vi "CSM User Interface(UI) Module Template.vi"(7 "Name (\"\" to Use UUID)":string="Event CSM") -> ()   [LabVIEW 2017]
doc: "A template for creating a CSM module with a user interface. This template includes a user Event Structure for responding to user actions.\n\n\n> [!NOTE] <b>CSM Naming Rules</b>\n>\n> - CSM module name must be unique. Otherwise, CSM enters a `Critical Error` state.\n> - If the input module name is an empty string (\"\"), the system uses a UUID as the module name. Such a module is marked as standalone mode and does not appear in the module list.\n> - Worker Mode Rule: If the input module name ends with `#`, a worker mode node will be instantiated. Multiple worker mode nodes can form a worker mode module.\n> - Chain of Responsibility Mode Rule: If the input module name ends with `$` followed by a number, a chain of responsibility mode node will be instantiated. Multiple chain of responsibility mode nodes can form a chain of responsibility mode module. Smaller numbers mean higher priority, and messages are routed directly to the highest-priority node that can handle them.\n> - System-Level Module Rule: If the input module name starts with `.`, the module is a system-level module. Under default settings, such modules are not listed by the CSM - List Modules VI and are suitable for instantiating modules that run in the background.\n> - Submodule Rule: `.` is also allowed in a module name to separate the module name into multiple parts. CSM does not have strict rules for submodules. The `.` in the module name only marks the logical relationship between different modules. From an execution perspective, they are considered independent modules. The only difference is that you can obtain a list of logical submodules via the CSM - List Submodules VI.\n\n\n> [!NOTE] <b>CSM Initialize State (\"Macro: Initialize\")</b>\n>\n> - The default value is `Macro: Initialize`, which is consistent with the JKISM state machine.\n> - This state is used to initialize the state machine of a CSM module. A CSM module will process externally sent messages only after completing this macro state.\n\n\n> [!NOTE] <b>CSM Exit State (\"Macro: Exit\")</b>\n>\n> - The default value is \"Macro: Exit\", which is consistent with the JKISM state machine.\n> - This state is used to exit the state machine of a CSM module. After entering this state, a CSM module no longer processes externally sent messages.\n\n\n> [!WARNING] <b>Multiple CSMs in a Single VI</b>\n>\n> - It is not recommended to place multiple (>=2) CSMs in a flat layout within a single VI. While this will not cause logical issues in the program, it will prevent the CSM Debug Console from loading all the inner and outer interfaces of the flat CSMs in that VI - only one will be loaded.\n\n\n-- <b>Controls</b> --\n- <b>Name (\"\" to use UUID)</b>: CSM module name. Refer to <b>CSM Naming Rules</b> for module naming rules."
uses:
  AdvanceAPI/CSM - Revert Arguments-Safe String.vi
  _Shared/Trim Single-line Text.vi
  AdvanceAPI/CSM - Break Down Multiple States String.vi
  AdvanceAPI/CSM - Compact Multiple States.vi
  AdvanceAPI/CSM - Make String Arguments Safe.vi
  AdvanceAPI/CSM - Keywords.vi
  Communicable State Machine.lvlib
panel:
  out "State History":string
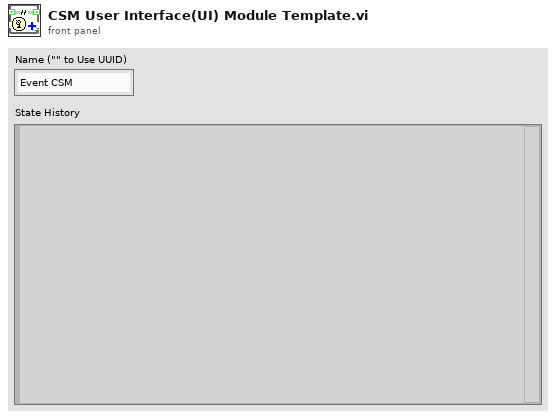
[diagram p1: front panel]
types:
  T1 = enum32{"Invalid", "Standard", "Closed", "Hidden", "Minimized", "Maximized"}
  T2 = enum32{"invalid app kind", "Development System", "Run Time System", "Student Edition", "Embedded LabVIEW", "Evaluation", "Custom"}
  T3 = typedef "Communicable State Machine.lvlib/_CSM_Response Source Message.ctl" = cluster{"‘State":string, "’Arguments":string, "’Error":errorcluster}
  T4 = cluster{"Current VI Reference":refnum<vi>, "Close Panel on Exit?":bool}
  T5 = cluster{"Core":cluster{"Current VI Reference":refnum<vi>, "Close Panel on Exit?":bool}, "Your Boolean data":bool, "Your string data":string}
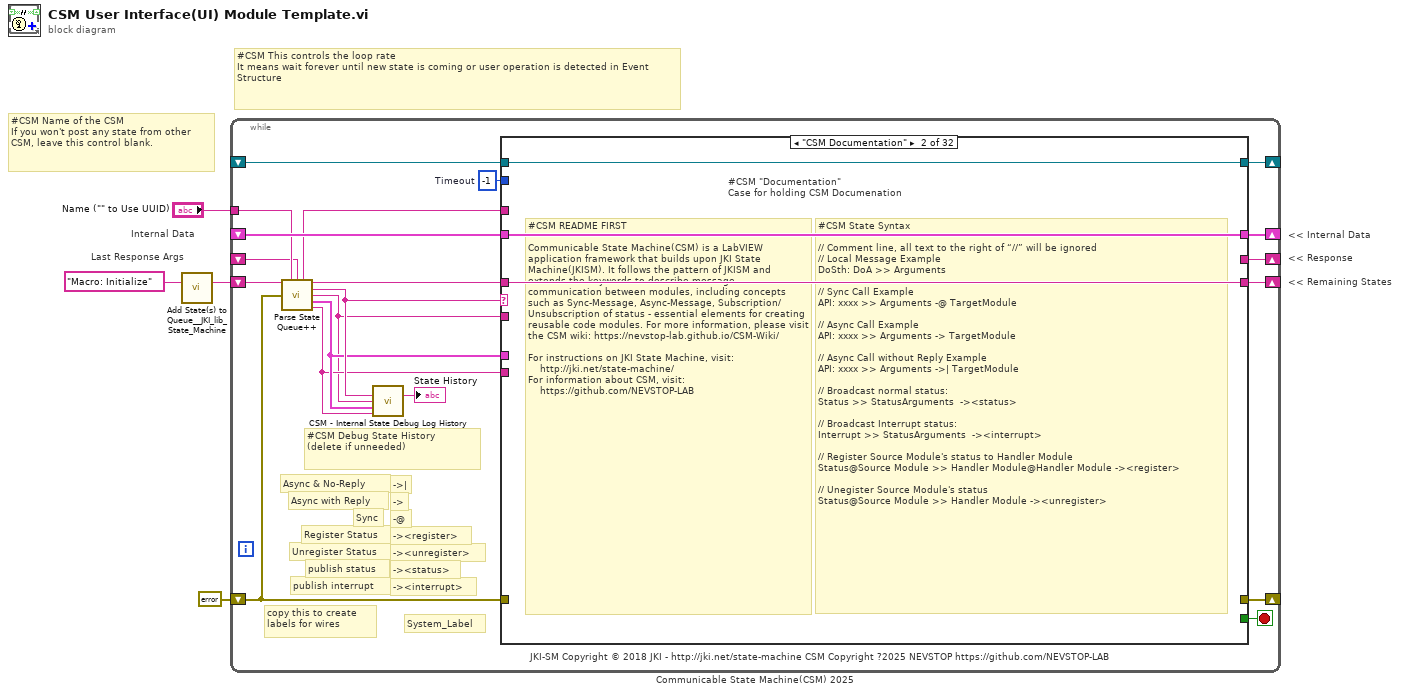
[diagram p0: block diagram]
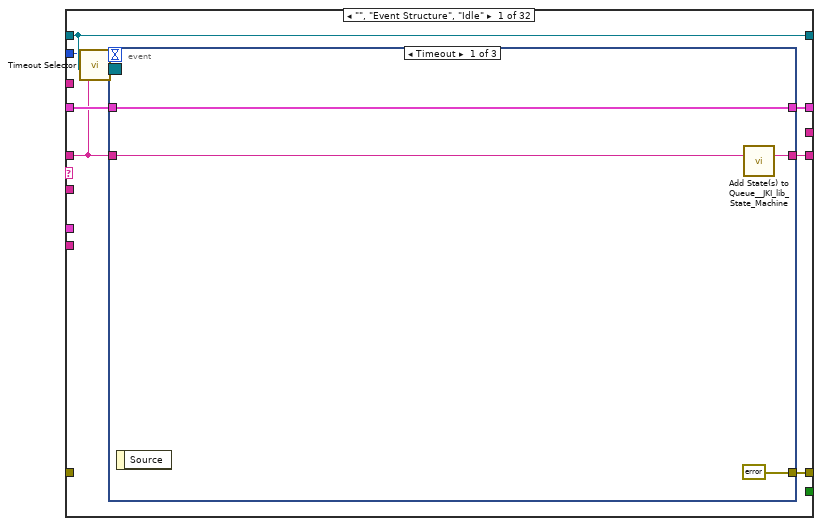
[diagram p2: hidden frame]
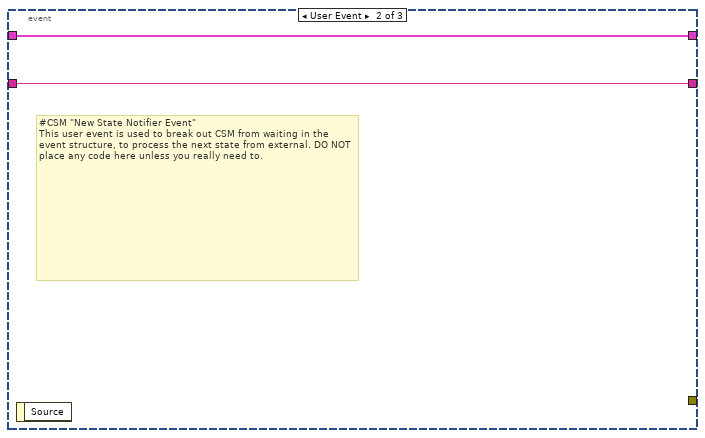
[diagram p3: hidden frame]
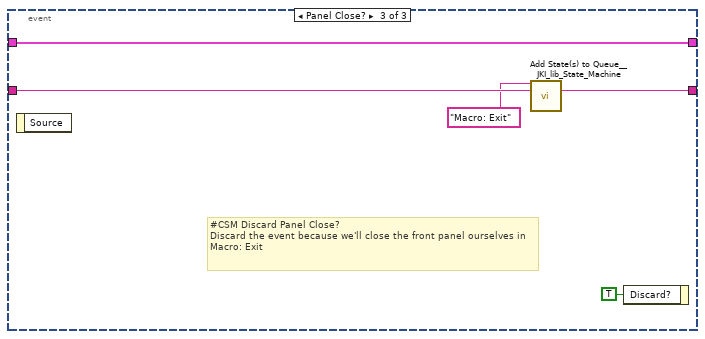
[diagram p4: hidden frame]
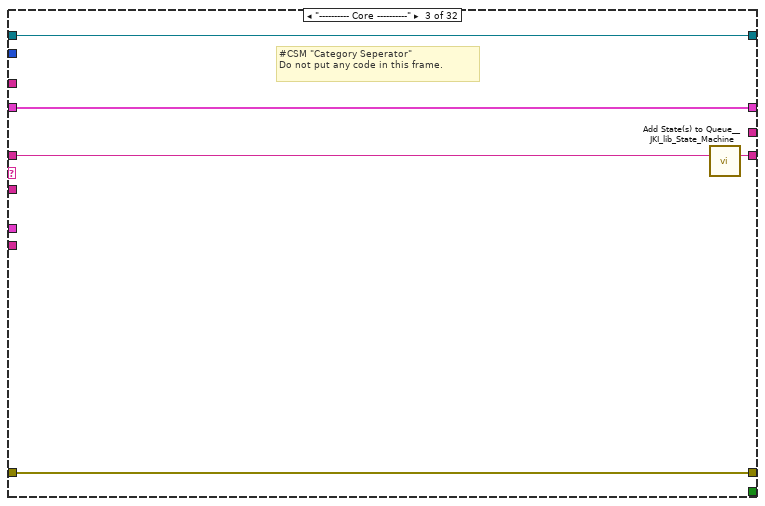
[diagram p5: hidden frame]
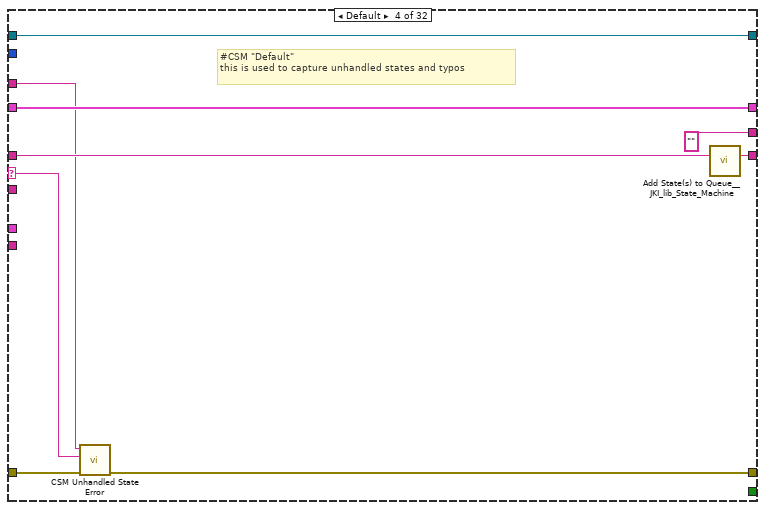
[diagram p6: hidden frame]
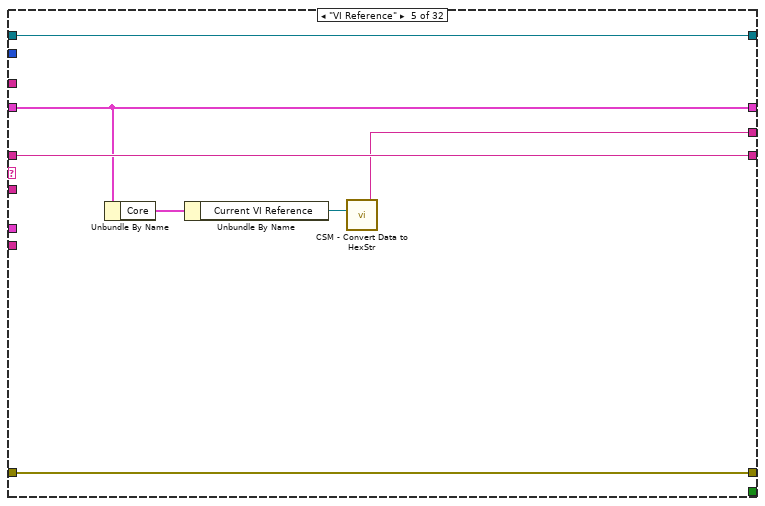
[diagram p7: hidden frame]
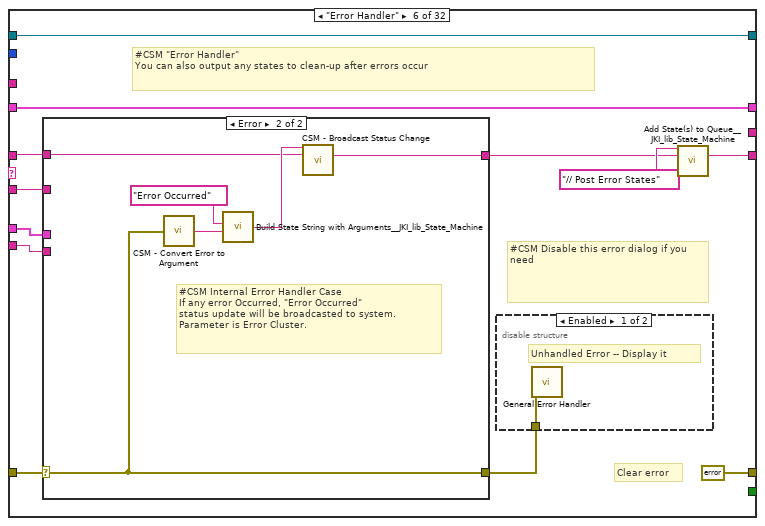
[diagram p8: hidden frame]
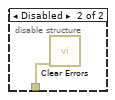
[diagram p9: hidden frame]
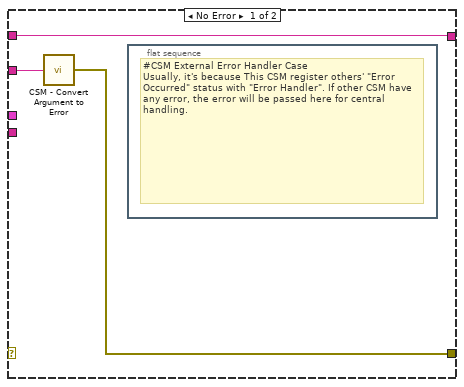
[diagram p10: hidden frame]
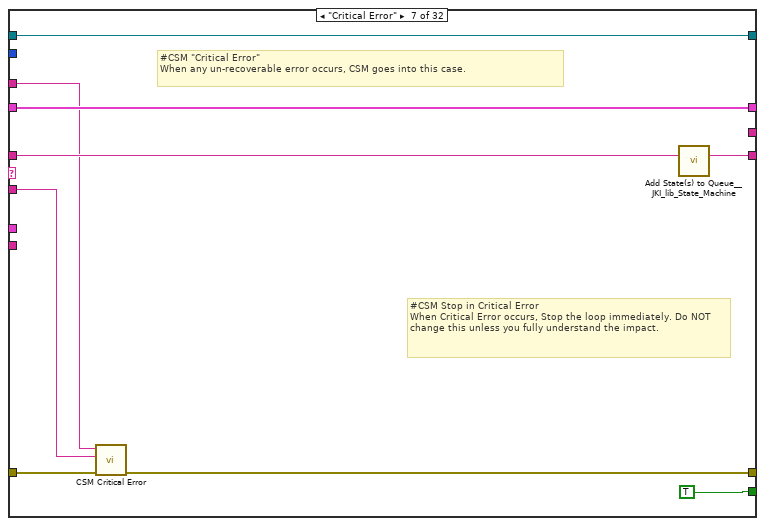
[diagram p11: hidden frame]
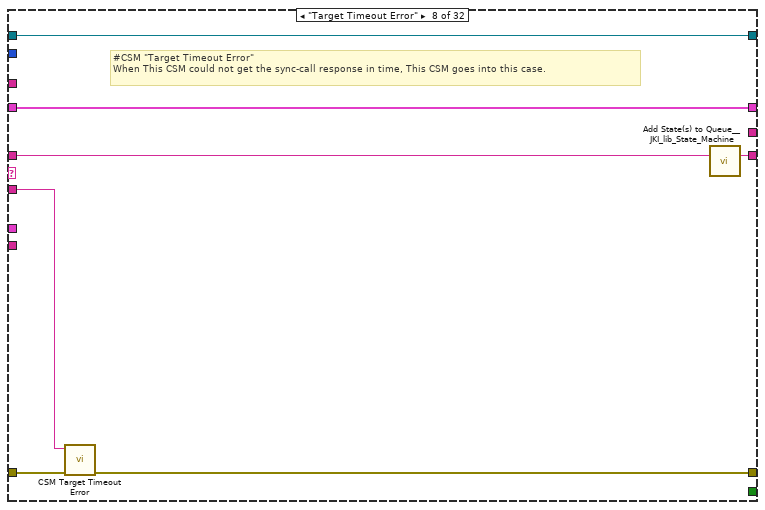
[diagram p12: hidden frame]
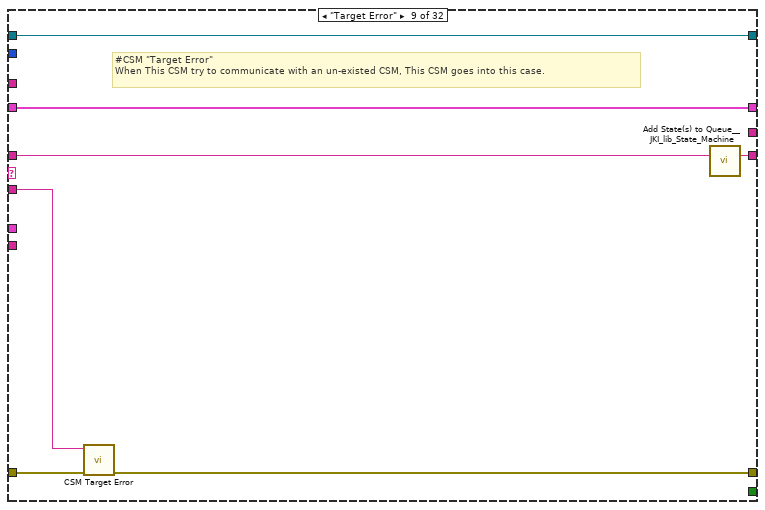
[diagram p13: hidden frame]
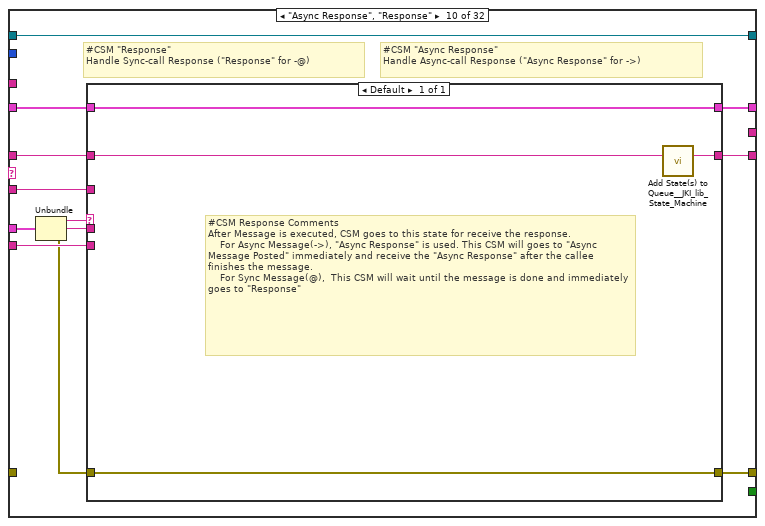
[diagram p14: hidden frame]
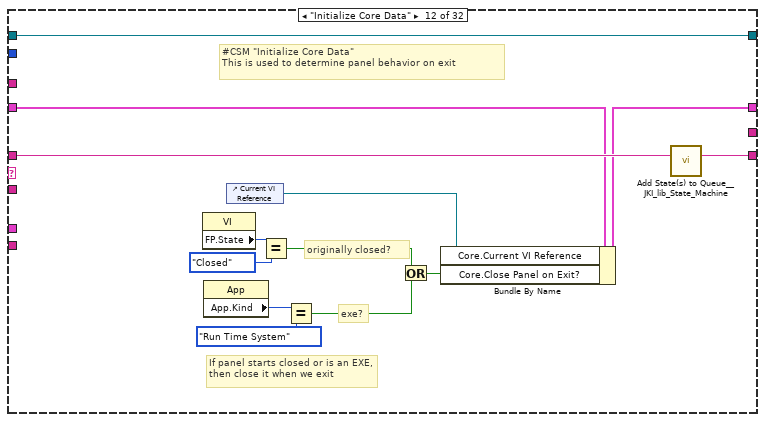
[diagram p16: hidden frame]
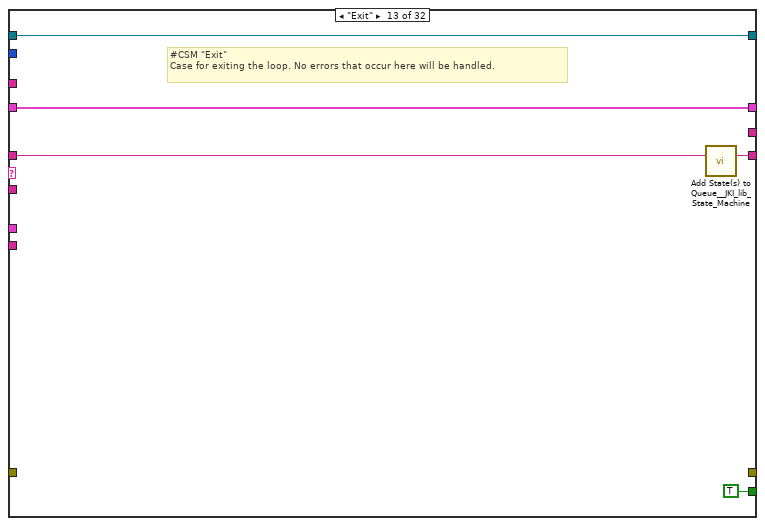
[diagram p17: hidden frame]
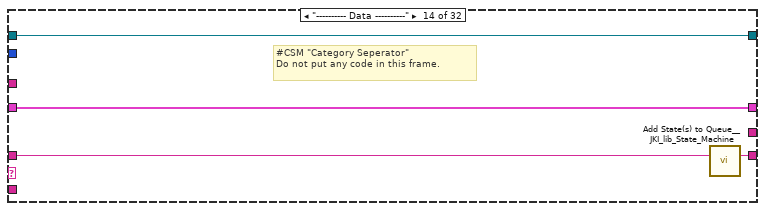
[diagram p18: hidden frame]
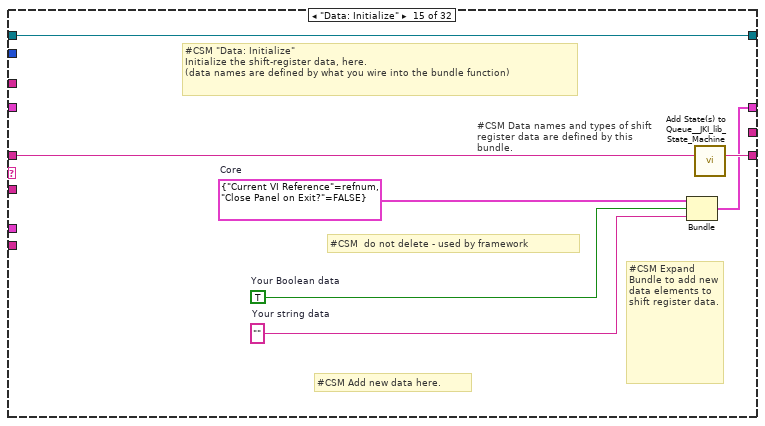
[diagram p19: hidden frame]
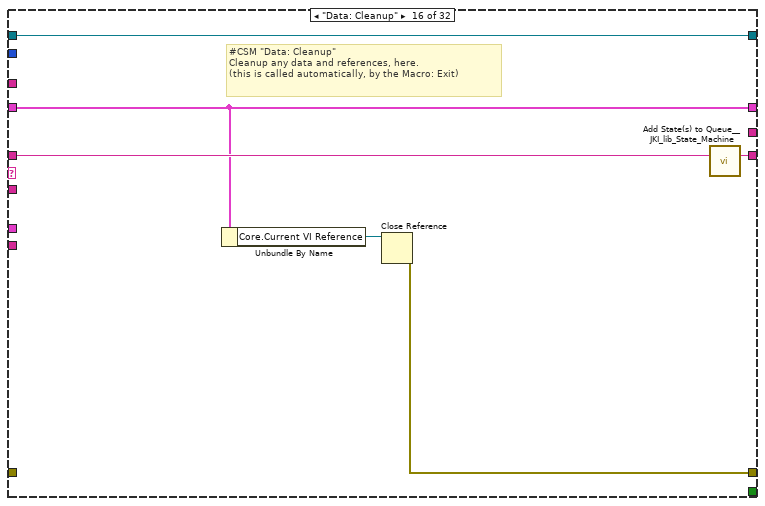
[diagram p20: hidden frame]
diagram:
  # "Last Response Args"
  # "Internal Data"
  # "<< Internal Data"
  # "<< Response"
  # "<< Remaining States"
  # "#CSM Name of the CSM\nIf you won't post any state from other CSM, leave this control blank."
  # "#CSM This controls the loop rate\nIt means wait forever until new state is coming or user operation is detected in Event Structure"
  n1 = call <vilib>:"Add State(s) to Queue__JKI_lib_State_Machine.vi"("State(s) in (\"\")"="Macro: Initialize" ("Init State(\"Macro: Initialize\")")) -> ("States Out"=w4:string)  [unwired: 14 in]
  n2 = while "Communicable State Machine(CSM) 2025" {
    shift-right: [w19] -> _
    shift-left: _ -> [w18]
    shift-right: [w22] -> _
    shift-left: errorcluster {"status"=FALSE, "code"=0, "source"=""} ("error out") -> [w16]
    shift-right: [w21] -> _
    shift-left: w4 -> [w23]
    tunnel: "Name (\"\" to Use UUID)" -> [w12]
    shift-right: [w15] -> _
    shift-left: _ -> [w7]
    shift-right: [w14] -> _
    shift-left: _ -> [w13]
    stop <- w20 stop-if-true
    w17 = -1  # Timeout
    # "#CSM Debug State History\n(delete if unneeded)"
    # "-><interrupt>"
    # "-><status>"
    # "-><unregister>"
    # "-><register>"
    # "-@"
    # "->"
    # "->|"
    # "publish interrupt"
    # "publish status"
    # "Unregister Status"
    # "Register Status"
    # "Sync"
    # "Async with Reply"
    # "Async & No-Reply"
    # "copy this to create labels for wires"
    # "System_Label"
    # "JKI-SM Copyright © 2018 JKI - http://jki.net/state-machine CSM Copyright ?2025 NEVSTOP https://github.com/NEVSTOP-LAB"
    n3 = call "Parse State Queue++.vi"("State Queue"=w23, "Name (\"\" to Use UUID)"=w12, "Response Arguments"=w7, "Previous Error"=w16) -> ("Name Used"=w8:string, "Remaining States"=w24:string, "Current State"=w11:string, "Arguments"=w6:string, "Additional Information"=w10:T3, "Source CSM"=w9:string)  [unwired: 6 in]
    n4 = call "CSM - Internal State Debug Log History.vi"("State"=w11, "Arguments (\"\")"=w6, ">> Response Source Message >>"=w10, "Source (\"\")"=w9) -> ("Debug Log"=→"State History":string)  [unwired: 11 in]
    n5 = case shown="\"CSM Documentation\"" w11 {
      selector: w11 -> [_ _ _ w54 _ _ _ _ _ _ _ _ _ _ _ _ _ _ _ _ _ _ _ _ _ _ _ _ _ _ _ _]
      tunnel: w24 -> [w25 w46 w51 w60 w66 w72 w98 w106 w113 w123 w132 w145 w150 w154 w161 w167 w171 w178 w182 w186 w190 w196 w207 w271 w276 w287 w290 w294 w297 w301 w305 w309]
      tunnel: w6 -> [_ _ _ _ _ w70 w94 w101 w109 w117 _ _ _ _ _ _ _ _ _ _ _ w192 w202 _ _ _ _ _ _ _ _ _]
      tunnel: w18 -> [w31 w45 w48 w58 w65 w78 w99 w104 w111 w121 w131 w139 w148 w152 _ w163 w169 w177 w181 w184 w188 w194 w204 w269 w274 w285 w289 w293 w296 w299 w303 w307]
      tunnel: [w30 _ w49 w52 w67 errorcluster {"status"=FALSE, "code"=0, "source"=""} ("error out") w91 w100 w107 w120 _ _ _ _ _ w164 _ w172 w180 _ _ w193 w205 _ _ _ _ _ _ _ _ _] -> w22
      tunnel: w16 -> [_ _ w49 w53 w67 w76 w92 w102 w108 _ _ _ _ _ _ _ _ _ _ _ _ _ _ _ _ _ _ _ _ _ _ _]
      tunnel: [w32 w46 w50 w59 w66 w74 w97 w105 w112 w124 w132 w144 w149 w153 w160 w166 w170 w178 w182 w185 w189 w195 w206 w270 w275 w286 w290 w294 w297 w300 w304 w308] -> w21
      tunnel: [_ _ _ _ _ _ TRUE _ _ _ _ _ TRUE _ _ _ _ _ _ _ _ _ _ _ _ _ _ _ _ _ _ _] -> w20
      tunnel: [w29 w45 w48 w58 w65 w78 w99 w104 w111 w122 w131 w143 w148 w152 w159 w163 w169 w177 w181 w184 w188 w194 w204 w269 w274 w285 w289 w293 w296 w299 w303 w307] -> w19
      tunnel: w17 -> [w27 _ _ _ _ _ _ _ _ _ _ _ _ _ _ _ _ _ _ _ _ _ _ _ _ _ _ _ _ _ _ _]
      tunnel: w9 -> [_ _ _ _ _ w69 _ _ _ w118 _ _ _ _ _ _ _ _ _ _ _ _ _ _ _ _ _ _ _ _ _ _]
      tunnel: w10 -> [_ _ _ _ _ w68 _ _ _ w119 _ _ _ _ _ _ _ _ _ _ _ _ _ _ _ _ _ _ _ _ _ _]
      tunnel: [_ _ _ "" w61 _ _ _ _ _ _ _ _ _ _ _ _ _ _ _ _ _ _ _ _ _ _ "API1 Response" _ _ _ _] -> w15
      tunnel: [w28 w44 w47 w56 w64 w77 w95 w103 w110 w125 w130 w133 w146 w151 w155 w162 w168 w176 w179 w183 w187 w191 w201 w268 w272 w278 w288 w292 w295 w298 w302 w306] -> w14
      tunnel: w13 -> [w28 w44 w47 w56 w64 w77 w95 w103 w110 w125 w130 w133 w146 w151 w155 w162 w168 _ w179 w183 w187 w191 w201 w268 w272 w278 w288 w292 w295 w298 w302 w306]
      tunnel: w8 -> [_ _ _ w55 _ _ w93 _ _ _ _ _ _ _ _ _ _ w175 _ _ _ _ _ _ _ _ _ _ _ _ _ _]
      frame "", "Event Structure", "Idle" {
        n6 = call "Timeout Selector.vi"("Remaining States"=w25, "Timeout Expected"=w27) -> ("Timeout"=w26:i32)  [unwired: 5 in]
        n7 = event shown="[0] Timeout" {
          selector: w28 -> [_ _ _]
          dyn-events: _ -> [_ _ _]
          timeout: w26 -> [_ _ _]
          tunnel: w25 -> [w36 w37 w43]
          tunnel: [w35 w37 w42] -> w32
          tunnel: w31 -> [w34 w38 w41]
          tunnel: [errorcluster {"status"=FALSE, "code"=0, "source"=""} ("error out") _ _] -> w30
          tunnel: [w34 w38 w41] -> w29
          event Timeout {
            n8 = event-data() -> ()  [unwired: 1 in, 1 out]
            n9 = call <vilib>:"Add State(s) to Queue__JKI_lib_State_Machine.vi"("State(s) in (\"\")"=w36) -> ("States Out"=w35:string)  [unwired: 14 in]
          }
          event User Event {
            # "#CSM \"New State Notifier Event\"\nThis user event is used to break out CSM from waiting in the event structure, to process the next state from external. DO NOT place any code here unless you really need to."
            n10 = event-data() -> ()  [unwired: 1 in, 1 out]
          }
          event Panel Close? {
            # "#CSM Discard Panel Close?\nDiscard the event because we'll close the front panel ourselves in Macro: Exit"
            n11 = event-data() -> ()  [unwired: 1 in, 1 out]
            n12 = call <vilib>:"Add State(s) to Queue__JKI_lib_State_Machine.vi"("State(s) in Front (\"\")"="Macro: Exit", "State(s) in (\"\")"=w43) -> ("States Out"=w42:string)  [unwired: 13 in]
            n13 = event-data("Discard?"=TRUE) -> ()  [unwired: 1 in, 1 out]
          }
        }
      }
      frame "CSM Documentation" {
        # "#CSM State Syntax\n\n// Comment line, all text to the right of “//” will be ignored\n// Local Message Example\nDoSth: DoA >> Arguments\n\n// Sync Call Example\nAPI: xxxx >> Arguments -@ TargetModule\n\n// Async Call Example\nAPI: xxxx >> Arguments -> TargetModule\n\n// Async Call without Reply Example\nAPI: xxxx >> Arguments ->| TargetModule\n\n// Broadcast normal status:\nStatus >> StatusArguments  -><status>\n\n// Broadcast Interrupt status:\nInterrupt >> StatusArguments  -><interrupt>\n\n// Register Source Module's status to Handler Module\nStatus@Source Module >> Handler Module@Handler Module -><register>\n\n// Unegister Source Module's status\nStatus@Source Module >> Handler Module -><unregister>"
        # "#CSM README FIRST\n\nCommunicable State Machine(CSM) is a LabVIEW application framework that builds upon JKI State Machine(JKISM). It follows the pattern of JKISM and extends the keywords to describe message communication between modules, including concepts such as Sync-Message, Async-Message, Subscription/Unsubscription of status - essential elements for creating reusable code modules. For more information, please visit the CSM wiki: https://nevstop-lab.github.io/CSM-Wiki/\n\nFor instructions on JKI State Machine, visit: \n    http://jki.net/state-machine/\nFor information about CSM, visit: \n    https://github.com/NEVSTOP-LAB"
        # "#CSM \"Documentation\"\nCase for holding CSM Documenation"
      }
      frame "---------- Core ----------" {
        # "#CSM \"Category Seperator\"\nDo not put any code in this frame."
        n14 = call <vilib>:"Add State(s) to Queue__JKI_lib_State_Machine.vi"("State(s) in (\"\")"=w51) -> ("States Out"=w50:string)  [unwired: 14 in]
      }
      frame Default {
        # "#CSM \"Default\"\nthis is used to capture unhandled states and typos"
        n15 = call "CSM Unhandled State Error.vi"("error in (no error)"=w53, "Undefined State"=w54, "CSM Name"=w55) -> ("error out"=w52:errorcluster)  [unwired: 8 in]
        n16 = call <vilib>:"Add State(s) to Queue__JKI_lib_State_Machine.vi"("State(s) in (\"\")"=w60) -> ("States Out"=w59:string)  [unwired: 14 in]
      }
      frame "VI Reference" {
        n17 = Unbundle By Name(w65) -> ("Core"=w63:T4)
        n18 = Unbundle By Name(w63) -> ("Current VI Reference"=w62:refnum<vi>)
        n19 = call "CSM - Convert Data to HexStr.vi"("Variant"=w62) -> ("HEX String (0-9,A-F)"=w61:string)  [unwired: 8 in]
      }
      frame "Error Handler" {
        # "#CSM Disable this error dialog if you need"
        # "#CSM \"Error Handler\"\nYou can also output any states to clean-up after errors occur"
        # "Clear error"
        n20 = case shown="Error" w76 {
          selector: w76 -> [_ w85]
          tunnel: [w83 w87] -> w73
          tunnel: w72 -> [w83 w86]
          tunnel: [w82 w85] -> w71
          tunnel: w70 -> [w84 _]
          tunnel: w69 -> [_ _]
          tunnel: w68 -> [_ _]
          frame No Error {
            n21 = call "CSM - Convert Argument to Error.vi"("Argument"=w84) -> ("Error"=w82:errorcluster)  [unwired: 4 in]
            n22 = flat-sequence {
              frame #0 {
                # "#CSM External Error Handler Case\nUsually, it's because This CSM register others' \"Error Occurred\" status with \"Error Handler\". If other CSM have any error, the error will be passed here for central handling."
              }
            }
          }
          frame Error {
            # "#CSM Internal Error Handler Case \nIf any error Occurred, \"Error Occurred\" \nstatus update will be broadcasted to system.\nParameter is Error Cluster."
            n23 = call "CSM - Convert Error to Argument.vi"("Error"=w85) -> ("Argument"=w89:string)  [unwired: 4 in]
            n24 = call <vilib>:"Build State String with Arguments__JKI_lib_State_Machine.vi"("Arguments (\"\")"=w89, "State"="Error Occurred" ("Status with Arguments")) -> ("State with Arguments"=w88:string)  [unwired: 4 in]
            n25 = call "CSM - Broadcast Status Change.vi"("Status With Arguments"=w88, "State Queue"=w86) -> ("Remaining States"=w87:string)  [unwired: 13 in]
          }
        }
        n26 = disable-structure shown="Enabled" {
          disable-tunnel: w71 -> [w80 w81]
          frame Enabled {
            # "Unhandled Error -- Display it"
            n27 = call <vilib>:"General Error Handler.vi"("error in (no error)"=w80) -> ()  [unwired: 10 in, 5 out]
          }
          frame Disabled {
            n28 = call <vilib>:"Clear Errors.vi"("error in (no error)"=w81) -> ()  [unwired: 5 in, 2 out]
          }
        }
        n29 = call <vilib>:"Add State(s) to Queue__JKI_lib_State_Machine.vi"("State(s) in Front (\"\")"="// Post Error States", "State(s) in (\"\")"=w73) -> ("States Out"=w74:string)  [unwired: 13 in]
      }
      frame "Critical Error" {
        # "#CSM \"Critical Error\"\nWhen any un-recoverable error occurs, CSM goes into this case."
        # "#CSM Stop in Critical Error\nWhen Critical Error occurs, Stop the loop immediately. Do NOT change this unless you fully understand the impact."
        n30 = call "CSM Critical Error.vi"("error in (no error)"=w92, "Arugments (As Reason)"=w94, "CSM Name"=w93) -> ("error out"=w91:errorcluster)  [unwired: 8 in]
        n31 = call <vilib>:"Add State(s) to Queue__JKI_lib_State_Machine.vi"("State(s) in (\"\")"=w98) -> ("States Out"=w97:string)  [unwired: 14 in]
      }
      frame "Target Timeout Error" {
        # "#CSM \"Target Timeout Error\"\nWhen This CSM could not get the sync-call response in time, This CSM goes into this case."
        n32 = call "CSM Target Timeout Error.vi"("error in (no error)"=w102, "Arguments (As CSM Name)"=w101) -> ("error out"=w100:errorcluster)  [unwired: 9 in]
        n33 = call <vilib>:"Add State(s) to Queue__JKI_lib_State_Machine.vi"("State(s) in (\"\")"=w106) -> ("States Out"=w105:string)  [unwired: 14 in]
      }
      frame "Target Error" {
        # "#CSM \"Target Error\"\nWhen This CSM try to communicate with an un-existed CSM, This CSM goes into this case."
        n34 = call "CSM Target Error.vi"("error in (no error)"=w108, "Arguments (As CSM Name)"=w109) -> ("error out"=w107:errorcluster)  [unwired: 9 in]
        n35 = call <vilib>:"Add State(s) to Queue__JKI_lib_State_Machine.vi"("State(s) in (\"\")"=w113) -> ("States Out"=w112:string)  [unwired: 14 in]
      }
      frame "Async Response", "Response" {
        # "#CSM \"Async Response\"\nHandle Async-call Response (\"Async Response\" for ->)"
        # "#CSM \"Response\"\nHandle Sync-call Response (\"Response\" for -@)"
        n36 = Unbundle(w119) -> ("‘State"=w116:string, "’Arguments"=w115:string, "’Error"=w114:errorcluster)
        n37 = case shown="Default" w116 {
          tunnel: [w126] -> w124
          tunnel: w123 -> [w127]
          tunnel: [w129] -> w122
          tunnel: w121 -> [w129]
          tunnel: [w128] -> w120
          tunnel: w114 -> [w128]
          tunnel: w118 -> [_]
          tunnel: w117 -> [_]
          tunnel: w115 -> [_]
          frame Default {
            # "#CSM Response Comments\nAfter Message is executed, CSM goes to this state for receive the response.\n    For Async Message(->), \"Async Response\" is used. This CSM will goes to \"Async Message Posted\" immediately and receive the \"Async Response\" after the callee finishes the message.\n    For Sync Message(@),  This CSM will wait until the message is done and immediately goes to \"Response\""
            n38 = call <vilib>:"Add State(s) to Queue__JKI_lib_State_Machine.vi"("State(s) in (\"\")"=w127) -> ("States Out"=w126:string)  [unwired: 14 in]
          }
        }
      }
      frame "Async Message Posted" {
        # "#CSM \"Async Message Posted\"\nAfter Async Message is posted (-> or ->| ), CSM goes to this state for post-action.\nYou can use Argument - State to tell which Async Message is called."
      }
      frame "Initialize Core Data" {
        # "#CSM \"Initialize Core Data\"\nThis is used to determine panel behavior on exit"
        # "originally closed?"
        # "exe?"
        # "If panel starts closed or is an EXE, then close it when we exit"
        n39 = property class="VI"() -> ("FP.State"=w136:T1)  [unwired: 2 in, 2 out]
        n40 = property class="App"() -> ("App.Kind"=w142:T2)  [unwired: 2 in, 2 out]
        n41 = control-ref of="Current VI Reference"() -> (w137:refnum<vi>)
        n42 = Equal?(x=w136, y=T1."Closed" ("Front Panel Window:State")) -> (x = y?=w134:bool)
        n43 = Equal?(x=w142, y=T2."Run Time System" ("Application:Kind")) -> (x = y?=w140:bool)
        n44 = Or(x=w134, y=w140) -> (x .or. y?=w138:bool)
        n45 = Bundle By Name(cluster=w139, "Core.Current VI Reference"=w137, "Core.Close Panel on Exit?"=w138) -> (w143:T5)
        n46 = call <vilib>:"Add State(s) to Queue__JKI_lib_State_Machine.vi"("State(s) in (\"\")"=w145) -> ("States Out"=w144:string)  [unwired: 14 in]
      }
      frame "Exit" {
        # "#CSM \"Exit\"\nCase for exiting the loop. No errors that occur here will be handled."
        n47 = call <vilib>:"Add State(s) to Queue__JKI_lib_State_Machine.vi"("State(s) in (\"\")"=w150) -> ("States Out"=w149:string)  [unwired: 14 in]
      }
      frame "---------- Data ----------" {
        # "#CSM \"Category Seperator\"\nDo not put any code in this frame."
        n48 = call <vilib>:"Add State(s) to Queue__JKI_lib_State_Machine.vi"("State(s) in (\"\")"=w154) -> ("States Out"=w153:string)  [unwired: 14 in]
      }
      frame "Data: Initialize" {
        w156 = T4 {"Current VI Reference"=refnum, "Close Panel on Exit?"=FALSE}  # Core
        w158 = TRUE  # Your Boolean data
        w157 = ""  # Your string data
        # "#CSM  do not delete - used by framework"
        # "#CSM Expand Bundle to add new data elements to shift register data."
        # "#CSM Add new data here."
        # "#CSM Data names and types of shift register data are defined by this bundle."
        # "#CSM \"Data: Initialize\"\nInitialize the shift-register data, here.\n(data names are defined by what you wire into the bundle function)"
        n49 = Bundle("Core"=w156, "Your Boolean data"=w158, "Your string data"=w157) -> (w159:T5)  [unwired: 1 in]
        n50 = call <vilib>:"Add State(s) to Queue__JKI_lib_State_Machine.vi"("State(s) in (\"\")"=w161) -> ("States Out"=w160:string)  [unwired: 14 in]
      }
      frame "Data: Cleanup" {
        # "#CSM \"Data: Cleanup\"\nCleanup any data and references, here.\n(this is called automatically, by the Macro: Exit)"
        n51 = Unbundle By Name(w163) -> ("Core.Current VI Reference"=w165:refnum<vi>)
        n52 = Close Reference(reference=w165) -> (error out=w164:errorcluster)  [unwired: 1 in]
        n53 = call <vilib>:"Add State(s) to Queue__JKI_lib_State_Machine.vi"("State(s) in (\"\")"=w167) -> ("States Out"=w166:string)  [unwired: 14 in]
      }
      frame "---------- Events ----------" {
        # "#CSM \"Category Seperator\"\nDo not put any code in this frame."
        n54 = call <vilib>:"Add State(s) to Queue__JKI_lib_State_Machine.vi"("State(s) in (\"\")"=w171) -> ("States Out"=w170:string)  [unwired: 14 in]
      }
      frame "Events: Register" {
        # "#CSM \"Events: Register\"\nRegister user event. New Message Event is registered to break CSM waiting in event structure by default."
        # "#CSM Register New Message Event\nRegister message event to break Waiting in Event structure."
        n55 = call "CSM - Get New State Notifier Event.vi"("Name (\"\" to Use UUID)"=w175) -> ("error out"=w173:errorcluster, "New State Notifier Event"=w174:refnum<user-event>)  [unwired: 9 in]
        n56 = register-events(error in=w173, w174) -> (reference out=w176:refnum<event-registration>, error out=w172:errorcluster)  [unwired: 1 in]
      }
      frame "Events: Unregister" {
        # "#CSM \"Events: Unregister\"\nUnregister user event."
        n57 = Unregister For Events(event registration refnum=w179) -> (error out=w180:errorcluster)  [unwired: 1 in]
      }
      frame "---------- UI ----------" {
        # "#CSM \"Category Seperator\"\nDo not put any code in this frame."
        n58 = call <vilib>:"Add State(s) to Queue__JKI_lib_State_Machine.vi"("State(s) in (\"\")"=w186) -> ("States Out"=w185:string)  [unwired: 14 in]
      }
      frame "UI: Initialize" {
        # "#CSM \"UI: Initialize\"\nInitialize the User Interface, here.\n(this is called automatically, by the Macro: Init)"
        n59 = call <vilib>:"Add State(s) to Queue__JKI_lib_State_Machine.vi"("State(s) in (\"\")"=w190) -> ("States Out"=w189:string)  [unwired: 14 in]
      }
      frame "UI: Cursor Set" {
        # "Argument"
        # "#CSM \"UI: Cursor Set\"\nSet and Unset Cursor Busy.\n(Usage: \"UI: Cursor Set >> Busy|Idle\")"
        n60 = disable-structure shown="TARGET_TYPE!=Windows" {
          disable-tunnel: [w198 _] -> w193
          disable-tunnel: w192 -> [w197 _]
          frame condition #0 (active) {
            n61 = case shown="\"Idle\", Default" w197 {
              tunnel: [w199 w200] -> w198
              frame "Idle", Default {
                n62 = call <vilib>:"Unset Busy.vi"() -> ("error out"=w199:errorcluster)  [unwired: 11 in]
              }
              frame "Busy" {
                n63 = call <vilib>:"Set Busy.vi"() -> ("error out"=w200:errorcluster)  [unwired: 10 in, 1 out]
              }
            }
          }
          frame condition #1 {
          }
        }
        n64 = call <vilib>:"Add State(s) to Queue__JKI_lib_State_Machine.vi"("State(s) in (\"\")"=w196) -> ("States Out"=w195:string)  [unwired: 14 in]
      }
      frame "UI: Front Panel State" {
        # "Argument"
        # "#CSM \"UI: Front Panel State\"\nSet Front Panel Open or Closed\n(Usage: \"UI: Front Panel State >> Open|Close\")"
        n65 = Unbundle By Name(w204) -> ("Core.Current VI Reference"=w203:refnum<vi>)
        n66 = case shown="\"Minimize\", \"Minimized\"" w202 {
          tunnel: [w214 w227 w238 w250 w262] -> w205
          tunnel: w203 -> [w213 w225 w237 w249 w261]
          frame "Open", "Standard", Default {
            w208 = T1."Standard" ("State")
            n67 = property class="VI"(reference=w213) -> (reference out=w211:refnum<vi>, error out=w212:errorcluster, "FP.State"=w210:T1)  [unwired: 1 in]
            n68 = Not Equal?(x=w210, y=w208) -> (x != y?=w209:bool)
            n69 = case shown="True" w209 {
              tunnel: [w218 w220] -> w214
              tunnel: w212 -> [w217 w220]
              tunnel: w211 -> [w216 _]
              tunnel: w208 -> [w215 _]
              frame True {
                n70 = invoke class="VI" method="FP.Open"(reference=w216, error in=w217, "Activate"=TRUE, "State"=w215) -> (error out=w218:errorcluster)  [unwired: 1 in, 4 out]
              }
              frame False {
              }
            }
          }
          frame "Close", "Closed" {
            n71 = property class="VI"(reference=w225) -> (reference out=w224:refnum<vi>, error out=w226:errorcluster, "FP.State"=w222:T1)  [unwired: 1 in]
            n72 = Not Equal?(x=w222, y=T1."Closed" ("Front Panel Window:State")) -> (x != y?=w221:bool)
            n73 = case shown="True" w221 {
              tunnel: [w228 w231] -> w227
              tunnel: w226 -> [w228 w230]
              tunnel: w224 -> [_ w229]
              frame False {
              }
              frame True {
                n74 = invoke class="VI" method="FP.Close"(reference=w229, error in=w230) -> (error out=w231:errorcluster)  [unwired: 1 in, 2 out]
              }
            }
          }
          frame "Hidden", "Hide" {
            w232 = T1."Hidden" ("State")
            n75 = property class="VI"(reference=w237) -> (reference out=w235:refnum<vi>, error out=w236:errorcluster, "FP.State"=w234:T1)  [unwired: 1 in]
            n76 = Not Equal?(x=w234, y=w232) -> (x != y?=w233:bool)
            n77 = case shown="True" w233 {
              tunnel: [w242 w243] -> w238
              tunnel: w236 -> [w241 w243]
              tunnel: w235 -> [w240 _]
              tunnel: w232 -> [w239 _]
              frame True {
                n78 = invoke class="VI" method="FP.Open"(reference=w240, error in=w241, "State"=w239) -> (error out=w242:errorcluster)  [unwired: 2 in, 4 out]
              }
              frame False {
              }
            }
          }
          frame "Minimize", "Minimized" {
            w244 = T1."Minimized" ("State")
            n79 = property class="VI"(reference=w249) -> (reference out=w247:refnum<vi>, error out=w248:errorcluster, "FP.State"=w246:T1)  [unwired: 1 in]
            n80 = Not Equal?(x=w246, y=w244) -> (x != y?=w245:bool)
            n81 = case shown="False" w245 {
              tunnel: [w254 w255] -> w250
              tunnel: w248 -> [w253 w255]
              tunnel: w247 -> [w252 _]
              tunnel: w244 -> [w251 _]
              frame True {
                n82 = invoke class="VI" method="FP.Open"(reference=w252, error in=w253, "State"=w251) -> (error out=w254:errorcluster)  [unwired: 2 in, 4 out]
              }
              frame False {
              }
            }
          }
          frame "Maximize", "Maximized" {
            w256 = T1."Maximized" ("State")
            n83 = property class="VI"(reference=w261) -> (reference out=w259:refnum<vi>, error out=w260:errorcluster, "FP.State"=w258:T1)  [unwired: 1 in]
            n84 = Not Equal?(x=w258, y=w256) -> (x != y?=w257:bool)
            n85 = case shown="True" w257 {
              tunnel: [w266 w267] -> w262
              tunnel: w260 -> [w265 w267]
              tunnel: w259 -> [w264 _]
              tunnel: w256 -> [w263 _]
              frame True {
                n86 = invoke class="VI" method="FP.Open"(reference=w264, error in=w265, "State"=w263) -> (error out=w266:errorcluster)  [unwired: 2 in, 4 out]
              }
              frame False {
              }
            }
          }
        }
        n87 = call <vilib>:"Add State(s) to Queue__JKI_lib_State_Machine.vi"("State(s) in (\"\")"=w207) -> ("States Out"=w206:string)  [unwired: 14 in]
      }
      frame "---------- Macro ----------" {
        # "#CSM \"Category Seperator\"\nDo not put any code in this frame."
        n88 = call <vilib>:"Add State(s) to Queue__JKI_lib_State_Machine.vi"("State(s) in (\"\")"=w271) -> ("States Out"=w270:string)  [unwired: 14 in]
      }
      frame "Macro: Initialize" {
        w273 = "Data: Initialize\nInitialize Core Data\nEvents: Register\nUI: Initialize\nUI: Front Panel State >> Open"  # Data: Initialize Initialize Core Data Events: Register UI: Initialize UI: Front Panel State >> Open
        # "#CSM \"Macro: Initialize\"\nInitialization Macro (This is called once, when the VI starts)"
        n89 = call <vilib>:"Add State(s) to Queue__JKI_lib_State_Machine.vi"("State(s) in Front (\"\")"=w273, "State(s) in (\"\")"=w276) -> ("States Out"=w275:string)  [unwired: 13 in]
      }
      frame "Macro: Exit" {
        # "#CSM \"Macro: Exit\"\nExit Macro (This is called once, when the VI exits)"
        n90 = Unbundle By Name(w285) -> ("Core.Close Panel on Exit?"=w284:bool)
        n91 = Select(t="UI: Front Panel State >> Close", s=w284, f="") -> (s? t:f=w281:string)
        n92 = call <vilib>:"Add State(s) to Queue__JKI_lib_State_Machine.vi"("State(s) in Front (\"\")"="//Exit Sub-Modules ", "State(s) in (\"\")"=w281, "State(s) at Back (\"\")"="Data: Cleanup\nEvents: Unregister\nExit") -> ("States Out"=w279:string)  [unwired: 12 in]
        n93 = call <vilib>:"Add State(s) to Queue__JKI_lib_State_Machine.vi"("State(s) in Front (\"\")"=w279, "State(s) in (\"\")"=w287) -> ("States Out"=w286:string)  [unwired: 13 in]
      }
      frame "---------- API ----------" {
        # "#CSM \"Category Seperator\"\nDo not put any code in this frame."
      }
      frame "API: API1" {
        # "#CSM >> Source CSM >>\nIf you need to tell who triggered this state , use this string. If it's this case itself, this string is \"\"."
        # "#CSM >> Arguments >>\nDeal with the parameter if any"
        # "#CSM Response\nConnect this to return the response of your API"
        # "#CSM API Example\nCopy/Rename this case for your own API"
      }
      frame "API: API2" {
        # "#CSM API Example\nCopy/Rename this case for your own API"
      }
      frame "---------- Action ----------" {
        # "#CSM \"Category Seperator\"\nDo not put any code in this frame."
        n94 = call <vilib>:"Add State(s) to Queue__JKI_lib_State_Machine.vi"("State(s) in (\"\")"=w301) -> ("States Out"=w300:string)  [unwired: 14 in]
      }
      frame "Action: action1" {
        # "#CSM \"Internal State\"\nThis category is used for holding internal states"
        n95 = call <vilib>:"Add State(s) to Queue__JKI_lib_State_Machine.vi"("State(s) in (\"\")"=w305) -> ("States Out"=w304:string)  [unwired: 14 in]
      }
      frame "Action: action2" {
        # "#CSM \"Internal State\"\nThis category is used for holding internal states"
        n96 = call <vilib>:"Add State(s) to Queue__JKI_lib_State_Machine.vi"("State(s) in (\"\")"=w309) -> ("States Out"=w308:string)  [unwired: 14 in]
      }
    }
  }
